vi "Filter Thresholds (fast).vi"(7 "Thresholds":cluster{"Minimum":dbl, "Maximum":dbl}, 11 "Sorted Array":dbl[](array[numeric])) -> (3 "Filtered Array":dbl[](array[numeric]))   [LabVIEW 2018, in "Video Processor.lvclass"]
uses:
  Video Processor.lvclass
  3e917734-59b2-4db5-bda1-130cfc8f270d.vi
  de675af7-858c-41b1-81af-51575e7c3793.vi
  3e917734-59b2-4db5-bda1-130cfc8f270d.vi/ea80a8fa-701e-4cef-bef1-0767174e55f1.vi
  de675af7-858c-41b1-81af-51575e7c3793.vi/63c35067-443a-43e2-a5b8-027d34dc1bdc.vi
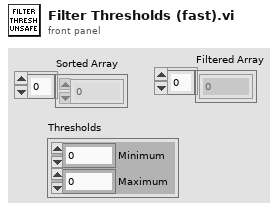
[diagram p1: front panel]
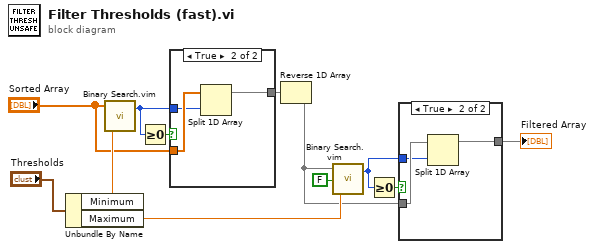
[diagram p0: block diagram]
diagram:
  n1 = Unbundle By Name("Thresholds") -> ("Minimum"=w11:dbl, "Maximum"=w7:dbl)
  n2 = call "Binary Search.vim"("Element"=w11, "Array"="Sorted Array") -> ("Index"=w3:i32)  [unwired: 1 in, 1 out]
  n3 = Greater Or Equal To 0?(x=w3) -> (x >= 0?=w4:bool)
  n4 = case shown="True" w4 {
    tunnel: w3 -> [_ w15]
    tunnel: "Sorted Array" -> [w13 w16]
    tunnel: [w13 w14] -> w9
    frame False {
    }
    frame True {
      n5 = Split 1D Array(array=w16, index=w15) -> (first subarray=w14:dbl[])  [unwired: 1 out]
    }
  }
  n6 = Reverse 1D Array(array=w9) -> (reversed array=w6:dbl[])
  n7 = call "Binary Search.vim"("Element"=w7, "Descending Order?"=FALSE, "Array"=w6) -> ("Index"=w1:i32)  [unwired: 1 out]
  n8 = Greater Or Equal To 0?(x=w1) -> (x >= 0?=w2:bool)
  n9 = case shown="True" w2 {
    tunnel: w1 -> [_ w19]
    tunnel: w6 -> [w17 w20]
    tunnel: [w17 w18] -> w5
    frame False {
    }
    frame True {
      n10 = Split 1D Array(array=w20, index=w19) -> (first subarray=w18:dbl[])  [unwired: 1 out]
    }
  }
  "Filtered Array" <- w5
